vi "Set Progressbar Color.vi"(10 "Progress bar Ref":refnum<vi>, 11 "Results":T1) -> (3 "Fill Color":u32(colorbox)=13840175)   [LabVIEW 2020, in "Execution UI.lvclass"]
uses:
  Execution UI.lvclass
  Result Model/Statistics.ctl
  Execution UI.lvclass/Execution UI.ctl
  Result Model/Result Model.lvclass
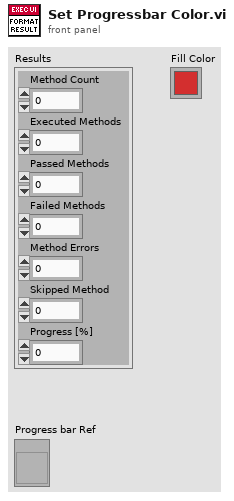
[diagram p1: front panel]
types:
  T1 = typedef "Result Model.lvclass/Statistics.ctl" = cluster{"Method Count":u32, "Executed Methods":u32, "Passed Methods":u32, "Failed Methods":u32, "Method Errors":u32, "Skipped Method":u32, "Progress [%]":dbl}
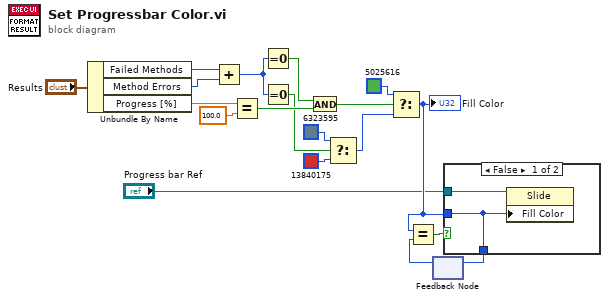
[diagram p0: block diagram]
diagram:
  n1 = Unbundle By Name("Results") -> ("Failed Methods"=w16:u32, "Method Errors"=w15:u32, "Progress [%]"=w18:dbl)
  n2 = Add(x=w16, y=w15) -> (x+y=w10:u32)
  n3 = Equal?(x=w18, y=100.0) -> (x = y?=w14:bool)
  n4 = Equal To 0?(x=w10) -> (x = 0?=w13:bool)
  n5 = Equal To 0?(x=w10) -> (x = 0?=w9:bool)
  n6 = And(x=w13, y=w14) -> (x .and. y?=w12:bool)
  n7 = Select(t=u32 6323595 ("Fill Color"), s=w9, f=u32 13840175 ("Fill Color")) -> (s? t:f=w6:u32)
  n8 = Select(t=u32 5025616 ("Fill Color"), s=w12, f=w6) -> (s? t:f=w2:u32)
  "Fill Color" <- w2
  n9 = feedback #1() -> (w5:u32)  [unwired: 1 in]
  n10 = Equal?(x=w2, y=w5) -> (x = y?=w4:bool)
  n11 = case shown="False" w4 {
    tunnel: w2 -> [w20 w22]
    tunnel: [w20 w22] -> w3
    tunnel: "Progress bar Ref" -> [w21 _]
    frame False {
      n12 = property on="Property Node" class="Slide"(reference=w21, "Fill Color"=w20) -> ()  [unwired: 1 in, 2 out]
    }
    frame True {
    }
  }
  n13 = feedback-in #1(w3) -> ()
